vi "Intake Mode Selector.vi"(9 "Manual":bool, 10 "Auto":bool) -> (2 "Intake Mode":T1)   [LabVIEW 2016]
uses:
  Common Code/Intake Modes.ctl
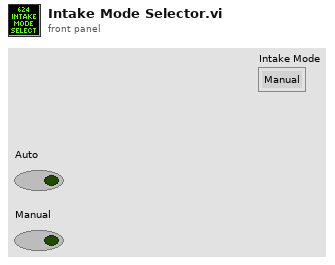
[diagram p1: front panel]
types:
  T1 = typedef "Intake Modes.ctl" = enum16{"Manual", "Auto"}
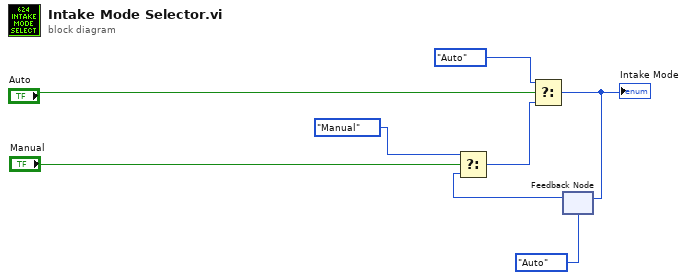
[diagram p0: block diagram]
diagram:
  n1 = feedback #1(Intake_Modes."Auto" ("Intake Modes")) -> (w1:T1)
  n2 = Select(t=Intake_Modes."Manual" ("Intake Modes"), s="Manual", f=w1) -> (s? t:f=w4:T1)
  n3 = Select(t=Intake_Modes."Auto" ("Intake Modes"), s="Auto", f=w4) -> (s? t:f=w2:T1)
  "Intake Mode" <- w2
  n4 = feedback-in #1(w2) -> ()
